vi "OP500InitParam_P.vi"(8 "errin":errorcluster, 11 "pathin":path) -> (0 "errout":errorcluster caption="error out")   [LabVIEW 2020]
uses:
  VG/VG_ISOmin_P.vi
  VG/VG_Conti.vi
  VG/VG_TenmaParam.vi
  ZEN8 Semi Auto EMC/OP700/VG/VG_TCellmin.vi
  ZEN8 Semi Auto EMC/OP700/VG/VG_TCellmax.vi
  VG/VG_TusineMin_P.vi
  VG/VG_TusineMax_P.vi
  VG/VG_VCellMin30_P.vi
  VG/VG_VCellMax30_P.vi
  VG/VG_VCellMin70_P.vi
  VG/VG_VCellMax70_P.vi
  VG/VG_DeltaTcell_P.vi
  VG/VG_DeltaVcell_P.vi
  VG/VG_DCIRmin_P.vi
  VG/VG_DCIRmax_P.vi
  VG/VG_OCV30max_P.vi
  VG/VG_OCV30min_P.vi
  VG/VG_OCV70max_P.vi
  VG/VG_OCV70min_P.vi
  VG/VG_DCIRCurrent_P.vi
  VG/VG_EquipementsNeeded_P.vi
  VG/VG_DCIR+OUIouNON_P.vi
  VG/VG_OP400_P.vi
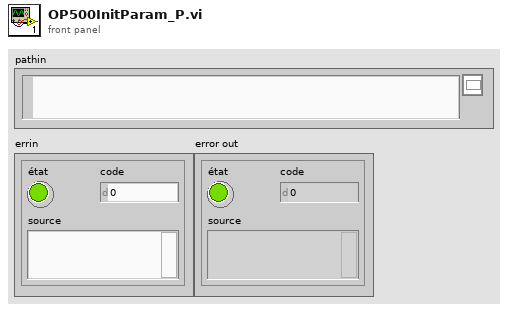
[diagram p1: front panel]
types:
  T1 = cluster{"[0]":dbl, "[1]":dbl, "[2]":dbl, "[3]":dbl, "[4]":dbl, "[5]":dbl, "[6]":dbl, "[7]":dbl, "[8]":dbl}
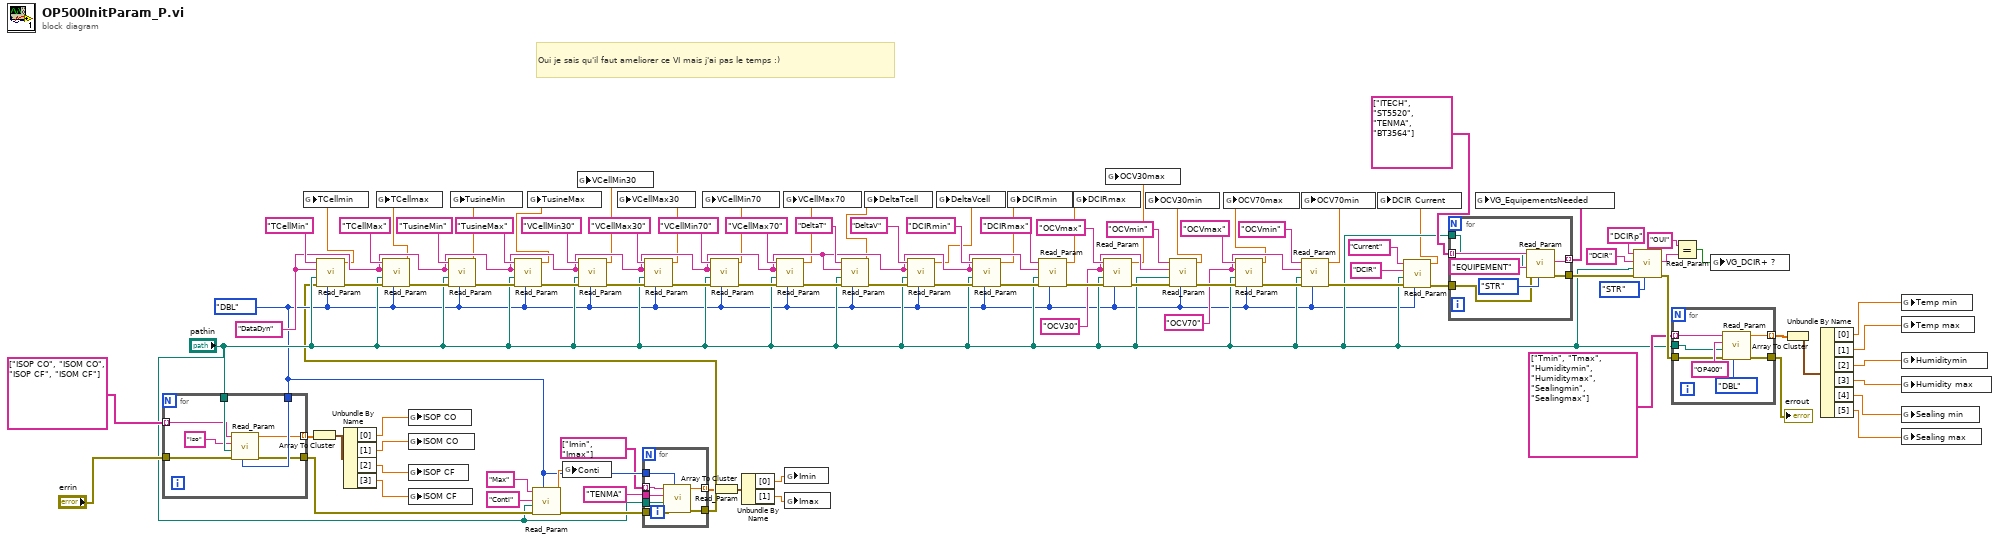
[diagram p0: block diagram]
diagram:
  w64 = "OCV70" ("section")
  w66 = "OCV30" ("section")
  w70 = "DataDyn" ("section")
  w9 = enum16{"STR", "DBL", "U32", "chemin"}."DBL" ("Énum")
  # "Oui je sais qu'il faut ameliorer ce VI mais j'ai pas le temps :)"
  n1 = for {
    tunnel: "errin" -> [w104]
    tunnel: w9 -> [w103]
    tunnel: "pathin" -> [w102]
    tunnel: string[] ["ISOP CO", "ISOM CO", "ISOP CF", "ISOM CF"] -> [w100] mode=indexing
    tunnel: [w99] -> w15
    tunnel: [w98] -> w21 mode=indexing
    n2 = call <userlib>:"Read_Param.vi"("Énum"=w103, "errin"=w104, "pathin"=w102, "section"="Iso", "key"=w100) -> ("error out"=w99:errorcluster, "dbl"=w98:dbl)  [unwired: 2 in, 3 out]
  }
  n3 = Array To Cluster(array=w21) -> (cluster=w20:T1)
  n4 = Unbundle By Name(w20) -> ("[0]"=w19:dbl, "[1]"=w18:dbl, "[2]"=w17:dbl, "[3]"=w16:dbl)
  n5 = global write "VG_ISOmin_P.vi" "ISOP CO"(w19) -> ()
  n6 = global write "VG_ISOmin_P.vi" "ISOM CO"(w18) -> ()
  n7 = global write "VG_ISOmin_P.vi" "ISOP CF"(w17) -> ()
  n8 = global write "VG_ISOmin_P.vi" "ISOM CF"(w16) -> ()
  n9 = call <userlib>:"Read_Param.vi"("Énum"=w9, "errin"=w15, "pathin"="pathin", "section"="Conti", "key"="Max") -> ("error out"=w11:errorcluster, "dbl"=w12:dbl)  [unwired: 2 in, 3 out]
  n10 = global write "VG_Conti.vi" "Conti"(w12) -> ()
  n11 = for {
    tunnel: w11 -> [w111]
    tunnel: "pathin" -> [w110]
    tunnel: w9 -> [w109]
    tunnel: "TENMA" ("section") -> [w108]
    tunnel: string[] ["Imin", "Imax"] -> [w107] mode=indexing
    tunnel: [w106] -> w6
    tunnel: [w105] -> w5 mode=indexing
    n12 = call <userlib>:"Read_Param.vi"("Énum"=w109, "errin"=w111, "pathin"=w110, "section"=w108, "key"=w107) -> ("error out"=w106:errorcluster, "dbl"=w105:dbl)  [unwired: 2 in, 3 out]
  }
  n13 = call <userlib>:"Read_Param.vi"("Énum"=w9, "errin"=w6, "pathin"="pathin", "section"=w70, "key"="TCellMin") -> ("error out"=w97:errorcluster, "dbl"=w63:dbl)  [unwired: 2 in, 3 out]
  n14 = global write "VG_TCellmin.vi" "TCellmin"(w63) -> ()
  n15 = call <userlib>:"Read_Param.vi"("Énum"=w9, "errin"=w97, "pathin"="pathin", "section"=w70, "key"="TCellMax") -> ("error out"=w96:errorcluster, "dbl"=w62:dbl)  [unwired: 2 in, 3 out]
  n16 = global write "VG_TCellmax.vi" "TCellmax"(w62) -> ()
  n17 = call <userlib>:"Read_Param.vi"("Énum"=w9, "errin"=w96, "pathin"="pathin", "section"=w70, "key"="TusineMin") -> ("error out"=w95:errorcluster, "dbl"=w61:dbl)  [unwired: 2 in, 3 out]
  n18 = global write "VG_TusineMin_P.vi" "TusineMin"(w61) -> ()
  n19 = call <userlib>:"Read_Param.vi"("Énum"=w9, "errin"=w95, "pathin"="pathin", "section"=w70, "key"="TusineMax") -> ("error out"=w94:errorcluster, "dbl"=w60:dbl)  [unwired: 2 in, 3 out]
  n20 = global write "VG_TusineMax_P.vi" "TusineMax"(w60) -> ()
  n21 = call <userlib>:"Read_Param.vi"("Énum"=w9, "errin"=w94, "pathin"="pathin", "section"=w70, "key"="VCellMin30") -> ("error out"=w93:errorcluster, "dbl"=w58:dbl)  [unwired: 2 in, 3 out]
  n22 = global write "VG_VCellMin30_P.vi" "VCellMin30"(w58) -> ()
  n23 = call <userlib>:"Read_Param.vi"("Énum"=w9, "errin"=w93, "pathin"="pathin", "section"=w70, "key"="VCellMax30") -> ("error out"=w92:errorcluster, "dbl"=w59:dbl)  [unwired: 2 in, 3 out]
  n24 = global write "VG_VCellMax30_P.vi" "VCellMax30"(w59) -> ()
  n25 = call <userlib>:"Read_Param.vi"("Énum"=w9, "errin"=w92, "pathin"="pathin", "section"=w70, "key"="VCellMin70") -> ("error out"=w91:errorcluster, "dbl"=w57:dbl)  [unwired: 2 in, 3 out]
  n26 = global write "VG_VCellMin70_P.vi" "VCellMin70"(w57) -> ()
  n27 = Array To Cluster(array=w5) -> (cluster=w4:T1)
  n28 = Unbundle By Name(w4) -> ("[0]"=w3:dbl, "[1]"=w2:dbl)
  n29 = call <userlib>:"Read_Param.vi"("Énum"=w9, "errin"=w91, "pathin"="pathin", "section"=w70, "key"="VCellMax70") -> ("error out"=w90:errorcluster, "dbl"=w56:dbl)  [unwired: 2 in, 3 out]
  n30 = global write "VG_VCellMax70_P.vi" "VCellMax70"(w56) -> ()
  n31 = global write "VG_TenmaParam.vi" "Imin"(w3) -> ()
  n32 = global write "VG_TenmaParam.vi" "Imax"(w2) -> ()
  n33 = call <userlib>:"Read_Param.vi"("Énum"=w9, "errin"=w90, "pathin"="pathin", "section"=w70, "key"="DeltaT") -> ("error out"=w89:errorcluster, "dbl"=w55:dbl)  [unwired: 2 in, 3 out]
  n34 = global write "VG_DeltaTcell_P.vi" "DeltaTcell"(w55) -> ()
  n35 = call <userlib>:"Read_Param.vi"("Énum"=w9, "errin"=w89, "pathin"="pathin", "section"=w70, "key"="DeltaV") -> ("error out"=w88:errorcluster, "dbl"=w42:dbl)  [unwired: 2 in, 3 out]
  n36 = global write "VG_DeltaVcell_P.vi" "DeltaVcell"(w42) -> ()
  n37 = call <userlib>:"Read_Param.vi"("Énum"=w9, "errin"=w88, "pathin"="pathin", "section"=w70, "key"="DCIRmin") -> ("error out"=w87:errorcluster, "dbl"=w54:dbl)  [unwired: 2 in, 3 out]
  n38 = global write "VG_DCIRmin_P.vi" "DCIRmin"(w54) -> ()
  n39 = call <userlib>:"Read_Param.vi"("Énum"=w9, "errin"=w87, "pathin"="pathin", "section"=w70, "key"="DCIRmax") -> ("error out"=w86:errorcluster, "dbl"=w53:dbl)  [unwired: 2 in, 3 out]
  n40 = global write "VG_DCIRmax_P.vi" "DCIRmax"(w53) -> ()
  n41 = call <userlib>:"Read_Param.vi"("Énum"=w9, "errin"=w86, "pathin"="pathin", "section"=w66, "key"="OCVmax") -> ("error out"=w85:errorcluster, "dbl"=w52:dbl)  [unwired: 2 in, 3 out]
  n42 = global write "VG_OCV30max_P.vi" "OCV30max"(w52) -> ()
  n43 = call <userlib>:"Read_Param.vi"("Énum"=w9, "errin"=w85, "pathin"="pathin", "section"=w66, "key"="OCVmin") -> ("error out"=w84:errorcluster, "dbl"=w51:dbl)  [unwired: 2 in, 3 out]
  n44 = global write "VG_OCV30min_P.vi" "OCV30min"(w51) -> ()
  n45 = call <userlib>:"Read_Param.vi"("Énum"=w9, "errin"=w84, "pathin"="pathin", "section"=w64, "key"="OCVmax") -> ("error out"=w83:errorcluster, "dbl"=w50:dbl)  [unwired: 2 in, 3 out]
  n46 = global write "VG_OCV70max_P.vi" "OCV70max"(w50) -> ()
  n47 = call <userlib>:"Read_Param.vi"("Énum"=w9, "errin"=w83, "pathin"="pathin", "section"=w64, "key"="OCVmin") -> ("error out"=w48:errorcluster, "dbl"=w49:dbl)  [unwired: 2 in, 3 out]
  n48 = global write "VG_OCV70min_P.vi" "OCV70min"(w49) -> ()
  n49 = call <userlib>:"Read_Param.vi"("Énum"=w9, "errin"=w48, "pathin"="pathin", "section"="DCIR", "key"="Current") -> ("error out"=w44:errorcluster, "dbl"=w1:dbl)  [unwired: 2 in, 3 out]
  n50 = global write "VG_DCIRCurrent_P.vi" "DCIR Current"(w1) -> ()
  n51 = for {
    tunnel: string[] ["ITECH", "ST5520", "TENMA", "BT3564"] -> [w118] mode=indexing
    tunnel: w44 -> [w115]
    tunnel: [w112] -> w41
    tunnel: [w114] -> w43 mode=indexing
    tunnel: "pathin" -> [w113]
    n52 = call <userlib>:"Read_Param.vi"("Énum"=enum16{"STR", "DBL", "U32", "chemin"}."STR", "errin"=w115, "pathin"=w113, "section"="EQUIPEMENT", "key"=w118) -> ("error out"=w112:errorcluster, "str"=w114:string)  [unwired: 2 in, 3 out]
  }
  n53 = global write "VG_EquipementsNeeded_P.vi" "VG_EquipementsNeeded"(w43) -> ()
  n54 = call <userlib>:"Read_Param.vi"("Énum"=enum16{"STR", "DBL", "U32", "chemin"}."STR", "errin"=w41, "pathin"="pathin", "section"="DCIR", "key"="DCIRp") -> ("error out"=w34:errorcluster, "str"=w37:string)  [unwired: 2 in, 3 out]
  n55 = for {
    tunnel: w34 -> [w124]
    tunnel: [w123] -> w33
    tunnel: string[] ["Tmin", "Tmax", "Humiditymin", "Humiditymax", "Sealingmin", "Sealingmax"] -> [w122] mode=indexing
    tunnel: "pathin" -> [w120]
    tunnel: [w119] -> w31 mode=indexing
    n56 = call <userlib>:"Read_Param.vi"("Énum"=enum16{"STR", "DBL", "U32", "chemin"}."DBL", "errin"=w124, "pathin"=w120, "section"="OP400", "key"=w122) -> ("error out"=w123:errorcluster, "dbl"=w119:dbl)  [unwired: 2 in, 3 out]
  }
  "errout" <- w33
  n57 = Equal?(x="OUI" ("key"), y=w37) -> (x = y?=w35:bool)
  n58 = global write "VG_DCIR+OUIouNON_P.vi" "VG_DCIR+ ?"(w35) -> ()
  n59 = Array To Cluster(array=w31) -> (cluster=w30:T1)
  n60 = Unbundle By Name(w30) -> ("[0]"=w29:dbl, "[1]"=w28:dbl, "[2]"=w27:dbl, "[3]"=w26:dbl, "[4]"=w25:dbl, "[5]"=w24:dbl)
  n61 = global write "VG_OP400_P.vi" "Temp min"(w29) -> ()
  n62 = global write "VG_OP400_P.vi" "Temp max"(w28) -> ()
  n63 = global write "VG_OP400_P.vi" "Humiditymin"(w27) -> ()
  n64 = global write "VG_OP400_P.vi" "Humidity max"(w26) -> ()
  n65 = global write "VG_OP400_P.vi" "Sealing min"(w25) -> ()
  n66 = global write "VG_OP400_P.vi" "Sealing max"(w24) -> ()
